vi "Write Numeric B.vi"(8 "error in (no error)":errorcluster, 10 "Abs_Types.lvlib:Numeric.lvclass":refnum<class "Abs_Numeric.lvclass">, 11 "Two Term SGL in":refnum<class "AbsFunc_Two Term_U16.lvclass">) -> (0 "error out":errorcluster, 3 "Two Term SGL out":refnum<class "AbsFunc_Two Term_U16.lvclass">)   [LabVIEW 2021, in "AbsFunc_Two Term_U16.lvclass"]
uses:
  AbsFunc_Two Term_U16.lvclass
  Abs_Types/Numeric/Abs_Numeric.lvclass
  AbsFunc_Two Term_U16.lvclass/AbsFunc_Two Term_U16.ctl
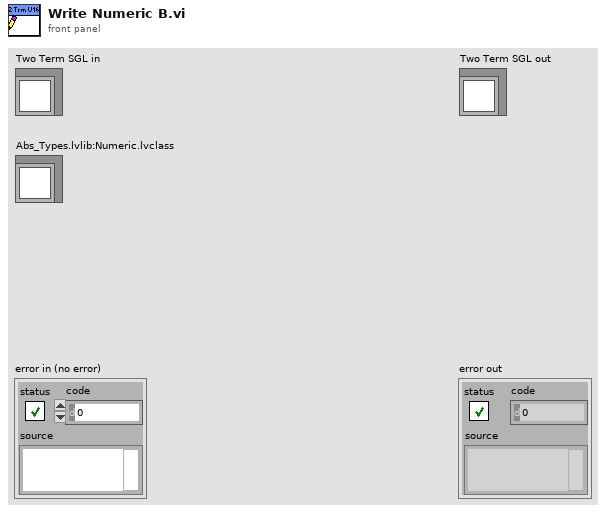
[diagram p1: front panel]
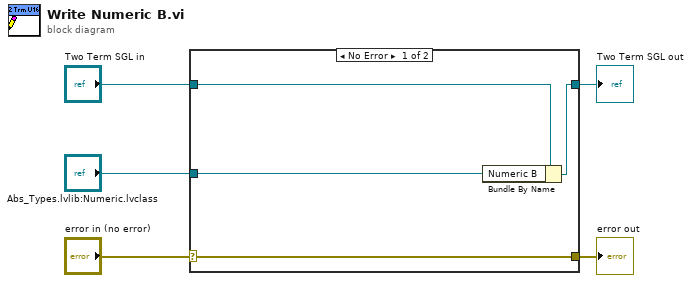
[diagram p0: block diagram]
diagram:
  n1 = case shown="No Error" "error in (no error)" {
    selector: "error in (no error)" -> [w9 w10]
    tunnel: [w9 w10] -> w4
    tunnel: [w7 w11] -> w2
    tunnel: "Two Term SGL in" -> [w8 w11]
    tunnel: "Abs_Types.lvlib:Numeric.lvclass" -> [w6 _]
    frame No Error {
      n2 = Bundle By Name(cluster=w8, "Numeric B"=w6) -> (w7:refnum<class "AbsFunc_Two Term_U16.lvclass">)
    }
    frame Error {
    }
  }
  "error out" <- w4
  "Two Term SGL out" <- w2
